vi "LoadController.vi"(8 "error in (no error)":errorcluster, 10 "Actor In":refnum<class "Actor.lvclass">, 11 "DemoLasers in":refnum<class "DemoLasers.lvclass">) -> (0 "error out":errorcluster, 3 "DemoLasers out":refnum<class "DemoLasers.lvclass">)   [LabVIEW 2020, in "DemoLasers.lvlib" / "DemoLasers.lvclass"]
uses:
  DemoLasers.lvclass
  <vilib>/ActorFramework/Actor/Actor.lvclass
  ViewController/OxxiusLaserController/OxxiusLaserController.lvclass
  C:/Program Files/National Instruments/LabVIEW 2020/vi.lib/ActorFramework/Actor/Actor.lvclass
  Hardware Abstraction Layer/Component/Laser/Laser/Laser.lvclass
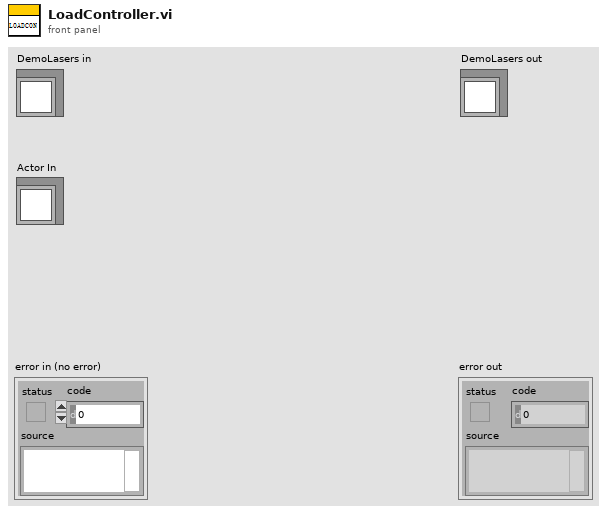
[diagram p1: front panel]
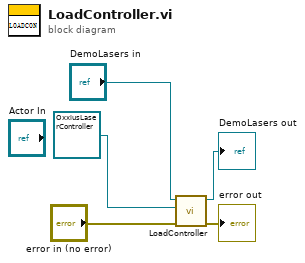
[diagram p0: block diagram]
diagram:
  n1 = call-parent "LoadController.vi"("error in (no error)"="error in (no error)", "Actor In"=refnum<class "OxxiusLaserController.lvclass"> refnum ("OxxiusLaserController.lvlib:OxxiusLaserController.lvclass"), "Device in"="DemoLasers in") -> ("error out"=→"error out":errorcluster, "Device out"=→"DemoLasers out":refnum<class "DemoLasers.lvclass">)  [unwired: 7 in]
